vi "SVXMPL_Configure Source.vi"(0 "acquisition task in":T5={"AI device settings"={"AI device"=1, "AI taskID"=0, "response"=[]}, "acquisition type"=enum."Finite", "measurement settings"={"AI sampling frequency"=51200.0, "AO sampling frequency"=51200.0, "AI block size"=1024, "AO block Size"=0, "block duration [ms]"=1024.0, "number of AI channels"=0, "board propagation time [samples]"=0, "DUT propagation time [s]"=0.0}, "settling settings"={"settle time"=0.015599999576807022, "settle cycles"=5}, "integration settings"={"integration time"=0.015599999576807022, "integration cycles"=5}, "AO device settings"={"AO device"=1, "AO taskID"=0, "excitation"=[]}, "acquisition accounting"={"initial read size [samples]"=0, "read offset [samples]"=0, "read length [samples]"=0, "blocks to settle [samples]"=0, "min delay until transition [samples]"=0}, "frequency range"={"start frequency"=0.015599999576807022, "stop frequency"=5.0}, "block type"=enum."Initialize", "source settings"={"signal type"=enum."Dual tone (IMD)", "frequency"=0.0, "total amplitude"=0.0, "frequencies"=[1.0], "relative amplitudes"=[1.0], "offset"=1.0, "total amplitude list"=[1.0], "ramping rate"=0.0}} {"source settings"."total amplitude" format="%.2f"; "source settings"."relative amplitudes" format="%.2f"; "source settings"."frequencies" format="%.2f"; "source settings"."total amplitude list" format="%.2f"; "source settings"."ramping rate" format="%.4f"; "source settings"."offset" format="%.2f"; "source settings"."frequency" format="%.2f"; "frequency range"."stop frequency" format="%.2f"; "frequency range"."start frequency" format="%.2f"; "AO device settings"."excitation"."output limits"."low limit (-10 V)" format="%.2f"; "AO device settings"."excitation"."output limits"."high limit (10 V)" format="%.2f"; "AI device settings"."response"."input limits"."low limit (0.0)" format="%.2f"; "AI device settings"."response"."input limits"."high limit (0.0)" format="%.2f"; "integration settings"."integration time" format="%.2p"; "settling settings"."settle time" format="%.2p"; "measurement settings"."DUT propagation time [s]" format="%.2f"; "measurement settings"."AO sampling frequency" format="%.2f"; "measurement settings"."AI sampling frequency" format="%.2f"}, 1 "signal type":T4(ring), 5 "sine frequency":dbl=1000.0 format="%.2f", 7 "total amplitude":dbl format="%.2f", 9 "amplitude-sweep amplitudes":dbl[](array[numeric]) format="%.2f", 11 "error in (no error)":errorcluster, 12 "IMD standard":T2(ring), 13 "custom IMD signal":T1={"IMD type"=enum."CCIF/Twin-Tone", "low-frequency tone"=14000.0, "high-frequency tone"=15000.0, "amplitude ratio"=1.0, "maximum order"=5} {"amplitude ratio" format="%.1f"; "high-frequency tone" format="%.2f"; "low-frequency tone" format="%.2f"}, 14 "multitone parameters":T3 {"component frequencies" format="%.2f"; "relative amplitudes" format="%.2f"}) -> (4 "acquisition task out":T5={"AI device settings"={"AI device"=1, "AI taskID"=0, "response"=[]}, "acquisition type"=enum."Finite", "measurement settings"={"AI sampling frequency"=51200.0, "AO sampling frequency"=51200.0, "AI block size"=1024, "AO block Size"=0, "block duration [ms]"=1024.0, "number of AI channels"=0, "board propagation time [samples]"=0, "DUT propagation time [s]"=0.0}, "settling settings"={"settle time"=0.015599999576807022, "settle cycles"=5}, "integration settings"={"integration time"=0.015599999576807022, "integration cycles"=5}, "AO device settings"={"AO device"=1, "AO taskID"=0, "excitation"=[]}, "acquisition accounting"={"initial read size [samples]"=0, "read offset [samples]"=0, "read length [samples]"=0, "blocks to settle [samples]"=0, "min delay until transition [samples]"=0}, "frequency range"={"start frequency"=0.015599999576807022, "stop frequency"=5.0}, "block type"=enum."Initialize", "source settings"={"signal type"=enum."Dual tone (IMD)", "frequency"=0.0, "total amplitude"=0.0, "frequencies"=[1.0], "relative amplitudes"=[1.0], "offset"=1.0, "total amplitude list"=[1.0], "ramping rate"=0.0}} {"source settings"."total amplitude" format="%.2f"; "source settings"."relative amplitudes" format="%.2f"; "source settings"."frequencies" format="%.2f"; "source settings"."total amplitude list" format="%.2f"; "source settings"."ramping rate" format="%.4f"; "source settings"."offset" format="%.2f"; "source settings"."frequency" format="%.2f"; "frequency range"."stop frequency" format="%.2f"; "frequency range"."start frequency" format="%.2f"; "AO device settings"."excitation"."output limits"."low limit (-10 V)" format="%.2f"; "AO device settings"."excitation"."output limits"."high limit (10 V)" format="%.2f"; "AI device settings"."response"."input limits"."low limit (0.0)" format="%.2f"; "AI device settings"."response"."input limits"."high limit (0.0)" format="%.2f"; "integration settings"."integration time" format="%.2p"; "settling settings"."settle time" format="%.2p"; "measurement settings"."DUT propagation time [s]" format="%.2f"; "measurement settings"."AO sampling frequency" format="%.2f"; "measurement settings"."AI sampling frequency" format="%.2f"}, 15 "error out":errorcluster)   [LabVIEW 2017]
doc: "This example VI allows you to configure the source that will be used for the synchronized AO/AI measurment.\n\nSet <B>signal type</B> to specify the nature of the excitation signal (e.g. whether the test signal is a sinewave, a multitone, a chirp, or noise).\n\nSet <B>total amplitude</B> to set the maximum amplitude of the time-domain excitation signal.\n\nOnly the source parameters associated with the selected signal type are configured."
uses:
  <vilib>/addons/Sound and Vibration/compatibility/Example Support/SVXMPL_Acquisition Task.ctl
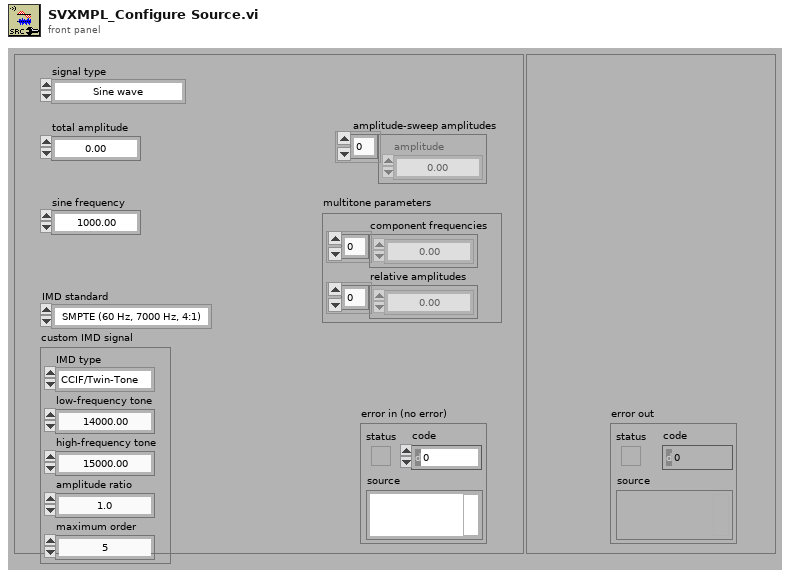
[diagram p1: front panel]
types:
  T1 = cluster{"IMD type":enum16{"SMPTE/DIN", "CCIF/Twin-Tone"}, "low-frequency tone":dbl, "high-frequency tone":dbl, "amplitude ratio":dbl, "maximum order":i32}
  T2 = enum16{"SMPTE (60 Hz, 7000 Hz, 4:1)", "DIN (250 Hz, 8000 Hz, 4:1)", "CCIF (11 kHz, 12 kHz, 1:1)", "CCIF (19 kHz, 20 kHz, 1:1)", "Custom"}
  T3 = cluster{"component frequencies":dbl[], "relative amplitudes":dbl[]}
  T4 = enum16{"Sine wave", "Dual tone (IMD)", "Multitone", "Chirp", "Frequency flat chirp", "Uniform white noise", "Gaussian white noise", "Pink noise", "PRN"}
  T5 = typedef "SVXMPL_Acquisition Task.ctl" = cluster{"AI device settings":cluster{"AI device":i16, "AI taskID":u32, "response":cluster{"AI channel":tag, "input limits":cluster{"high limit (0.0)":sgl, "low limit (0.0)":sgl}, "coupling & input config":cluster{"coupling":enum16{"no change", "DC", "AC", "GND", "internal ref."}, "input config":enum16{"no change", "differential", "ref. single-ended", "non-ref. single-ended", "4-wire"}}}[]}, "acquisition type":enum16{"Finite", "Averaged", "Settled", "Amplitude Sweep"}, "measurement settings":cluster{"AI sampling frequency":dbl, "AO sampling frequency":dbl, "AI block size":i32, "AO block Size":i32, "block duration [ms]":dbl, "number of AI channels":i32, "board propagation time [samples]":i32, "DUT propagation time [s]":dbl}, "settling settings":cluster{"settle time":dbl, "settle cycles":i32}, "integration settings":cluster{"integration time":dbl, "integration cycles":i32}, "AO device settings":cluster{"AO device":i16, "AO taskID":u32, "excitation":cluster{"AO Channel":tag, "output limits":cluster{"high limit (10 V)":sgl, "low limit (-10 V)":sgl, "reference source":enum16{"no change", "internal", "external"}}}[]}, "acquisition accounting":cluster{"initial read size [samples]":i32, "read offset [samples]":i32, "read length [samples]":i32, "blocks to settle [samples]":i32, "min delay until transition [samples]":i32}, "frequency range":cluster{"start frequency":dbl, "stop frequency":dbl}, "block type":enum16{"Initialize", "Settle", "Integrate"}, "source settings":cluster{"signal type":enum16{"Sine wave", "Dual tone (IMD)", "Multitone", "Chirp", "Frequency flat chirp", "Uniform white noise", "Gaussian white noise", "Pink noise", "PRN"}, "frequency":dbl, "total amplitude":dbl, "frequencies":dbl[], "relative amplitudes":dbl[], "offset":dbl, "total amplitude list":dbl[], "ramping rate":dbl}}
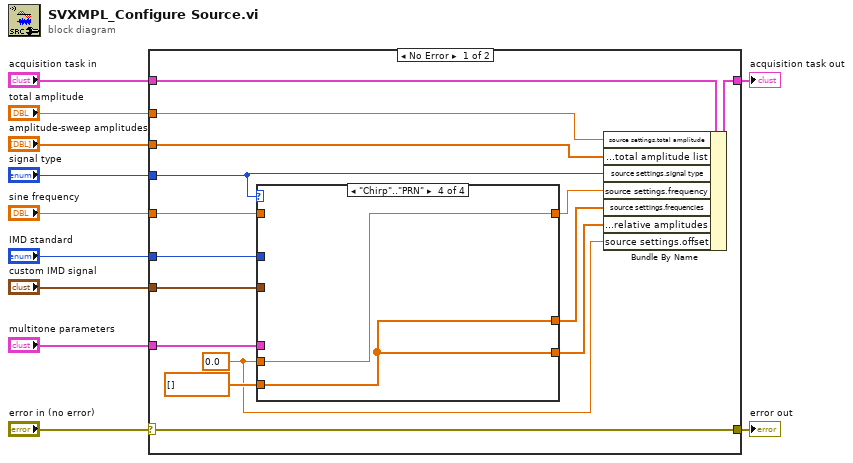
[diagram p0: block diagram]
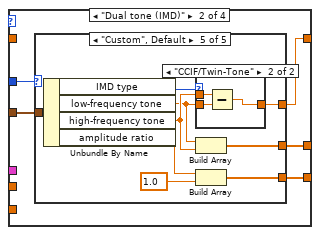
[diagram p3: hidden frame]
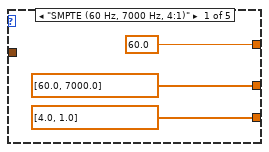
[diagram p4: hidden frame]
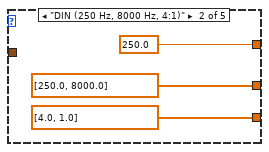
[diagram p5: hidden frame]
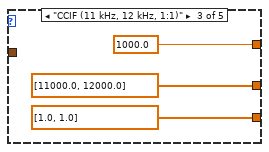
[diagram p6: hidden frame]
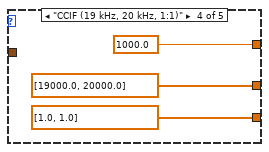
[diagram p7: hidden frame]
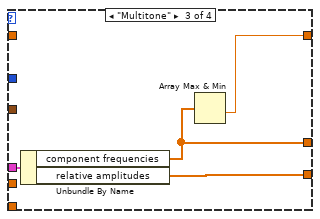
[diagram p9: hidden frame]
diagram:
  n1 = case shown="No Error" "error in (no error)" {
    selector: "error in (no error)" -> [w25 w66]
    tunnel: [w26 w65] -> w11
    tunnel: "acquisition task in" -> [w14 w65]
    tunnel: "signal type" -> [w16 _]
    tunnel: [w25 w66] -> w7
    tunnel: "amplitude-sweep amplitudes" -> [w15 _]
    tunnel: "custom IMD signal" -> [w23 _]
    tunnel: "multitone parameters" -> [w22 _]
    tunnel: "IMD standard" -> [w24 _]
    tunnel: "total amplitude" -> [w13 _]
    tunnel: "sine frequency" -> [w12 _]
    frame No Error {
      w19 = 0.0 ("amplitude")
      n2 = case shown="\"Chirp\"..\"PRN\"" w16 {
        tunnel: w23 -> [_ w32 _ _]
        tunnel: w22 -> [_ _ w62 _]
        tunnel: [w27 w29 w59 w64] -> w21
        tunnel: w19 -> [_ _ _ w64]
        tunnel: dbl[] [] ("source settings.frequencies") -> [w28 _ _ w63]
        tunnel: [w28 w30 w61 w63] -> w18
        tunnel: [w28 w31 w60 w63] -> w17
        tunnel: w24 -> [_ w33 _ _]
        tunnel: w12 -> [w27 _ _ _]
        frame "Sine wave", Default {
        }
        frame "Dual tone (IMD)" {
          n3 = case shown="\"Custom\", Default" w33 {
            tunnel: w32 -> [_ _ _ _ w54]
            tunnel: [dbl[] [60.0, 7000.0] ("source settings.frequencies") dbl[] [250.0, 8000.0] ("source settings.frequencies") dbl[] [11000.0, 12000.0] ("source settings.frequencies") dbl[] [19000.0, 20000.0] ("source settings.frequencies") w53] -> w31
            tunnel: [dbl[] [4.0, 1.0] ("source settings.frequencies") dbl[] [4.0, 1.0] ("source settings.frequencies") dbl[] [1.0, 1.0] ("source settings.frequencies") dbl[] [1.0, 1.0] ("source settings.frequencies") w52] -> w30
            tunnel: [60.0 ("low-frequency tone") 250.0 ("low-frequency tone") 1000.0 ("low-frequency tone") 1000.0 ("low-frequency tone") w46] -> w29
            frame "SMPTE (60 Hz, 7000 Hz, 4:1)" {
            }
            frame "DIN (250 Hz, 8000 Hz, 4:1)" {
            }
            frame "CCIF (11 kHz, 12 kHz, 1:1)" {
            }
            frame "CCIF (19 kHz, 20 kHz, 1:1)" {
            }
            frame "Custom", Default {
              n4 = Unbundle By Name(w54) -> ("IMD type"=w50:enum16{"SMPTE/DIN", "CCIF/Twin-Tone"}, "low-frequency tone"=w47:dbl, "high-frequency tone"=w48:dbl, "amplitude ratio"=w49:dbl)
              n5 = case shown="\"CCIF/Twin-Tone\"" w50 {
                tunnel: w48 -> [_ w58]
                tunnel: w47 -> [w55 w57]
                tunnel: [w55 w56] -> w46
                frame "SMPTE/DIN", Default {
                }
                frame "CCIF/Twin-Tone" {
                  n6 = Subtract(x=w58, y=w57) -> (x-y=w56:dbl)
                }
              }
              n7 = Build Array(w47, w48) -> (w53:dbl[])
              n8 = Build Array(w49, 1.0 ("element")) -> (w52:dbl[])
            }
          }
        }
        frame "Multitone" {
          n9 = Unbundle By Name(w62) -> ("component frequencies"=w60:dbl[], "relative amplitudes"=w61:dbl[])
          n10 = Array Max & Min(array=w60) -> (min value=w59:dbl)  [unwired: 3 out]
        }
        frame "Chirp".."PRN" {
        }
      }
      n11 = Bundle By Name(cluster=w14, "source settings.total amplitude"=w13, "source settings.total amplitude list"=w15, "source settings.signal type"=w16, "source settings.frequency"=w21, "source settings.frequencies"=w17, "source settings.relative amplitudes"=w18, "source settings.offset"=w19) -> (w26:T5)
    }
    frame Error {
    }
  }
  "acquisition task out" <- w11
  "error out" <- w7
